vi "Update VI List.vi"(10 "error in (no error)":errorcluster, 11 "Controller Array in":refnum<class "Controller Array.lvclass">) -> (2 "error out":errorcluster, 3 "Controller Array out":refnum<class "Controller Array.lvclass">)   [LabVIEW 2020, in "RxnRover.lvlib"]
doc: "Fires the Update VI List Event with the provided Controller Array."
uses:
  RxnRover.lvlib
  Plugin Servers/Controller Array/Controller Array.lvclass
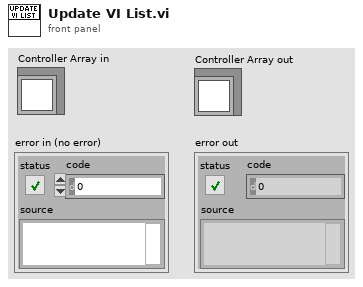
[diagram p1: front panel]
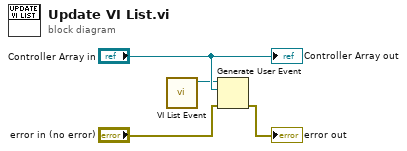
[diagram p0: block diagram]
diagram:
  n1 = call "VI List Event.vi"() -> ("VIs"=w3:refnum<user-event>)  [unwired: 11 in]
  n2 = Generate User Event(user event=w3, event data cluster="Controller Array in", error in="error in (no error)") -> (error out=→"error out":errorcluster)  [unwired: 1 in, 1 out]
  "Controller Array out" <- "Controller Array in"
